vi "CSM - All Relationships of Broadcast Registry.vi"() -> ()   [LabVIEW 2017, in "Communicable State Machine.lvlib"]
uses:
  Communicable State Machine.lvlib
  CSM - Broadcast Message Type.ctl
  _Support/FGV-BroadcastRegistry/global-CSMQ FGV Change Flag.vi
  _Support/CSMQ/_CSMOFGV.vi
panel:
  out "error out":errorcluster
  in  "error in (no error)":errorcluster
  out "Array":T2(array[cluster])
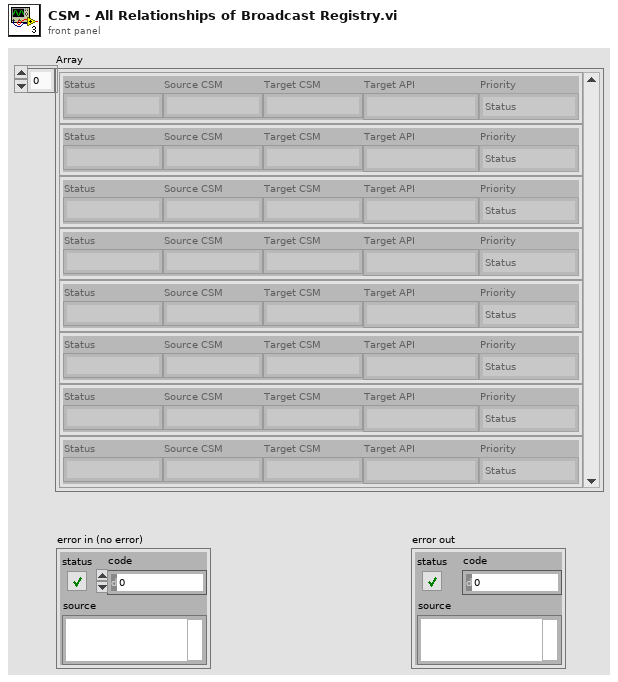
[diagram p1: front panel]
types:
  T1 = typedef "Communicable State Machine.lvlib/CSM - Broadcast Message Type.ctl" = enum16{"Status", "Interrupt(High)"}
  T2 = cluster{"Status":string, "Source CSM":string, "Target CSM":string, "Target API":string, "Priority":T1}[]
  T3 = cluster{"Target CSM":string, "Target State":string, "Priority":T1}[]
  T4 = cluster{"Status":string, "Source CSM":string, "Target CSM":string, "Target API":string, "Priority":T1}
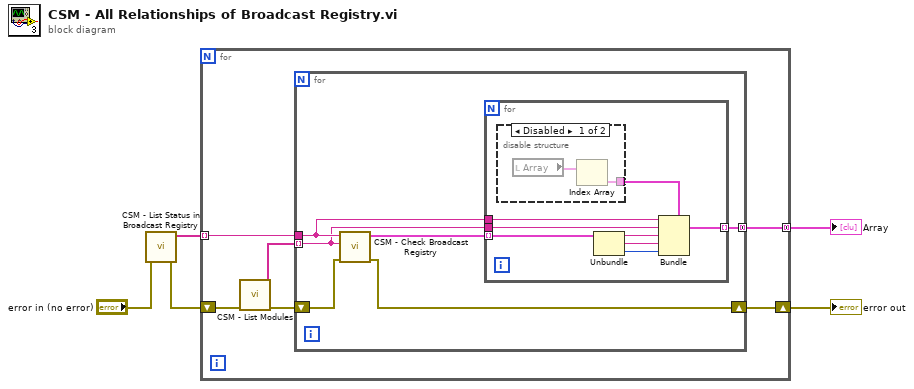
[diagram p0: block diagram]
diagram:
  n1 = call "CSM - List Status in Broadcast Registry.vi"("error in (no error)"="error in (no error)") -> ("error out"=w2:errorcluster, "Status in Registry"=w5:string[])  [unwired: 9 in]
  n2 = for {
    tunnel: w5 -> [w11] mode=indexing
    tunnel: [w9] -> w4 mode=concatenating
    shift-right: [w6] -> w1
    shift-left: w2 -> [w8]
    n3 = call "CSM - List Modules.vi"("Error in"=w8) -> ("Error out"=w7:errorcluster, "Module Names"=w10:string[])  [unwired: 9 in]
    n4 = for {
      tunnel: w11 -> [w17]
      tunnel: w10 -> [w15] mode=indexing
      tunnel: [w14] -> w9 mode=concatenating
      shift-right: [w12] -> w6
      shift-left: w7 -> [w13]
      n5 = call "CSM - Check Broadcast Registry.vi"("error in (no error)"=w13, "CSM Name"=w15, "Broadcast state"=w17) -> ("error out"=w12:errorcluster, "Array"=w16:T3)  [unwired: 7 in]
      n6 = for {
        tunnel: w17 -> [w25]
        tunnel: w16 -> [w22] mode=indexing
        tunnel: w15 -> [w24]
        tunnel: [w23] -> w14 mode=indexing
        n7 = disable-structure shown="Disabled" {
          disable-tunnel: [w26 _] -> w18
          frame Disabled {
            n8 = local read "Array"() -> (w27:T2)
            n9 = Index Array(array=w27) -> (element=w26:T4)  [unwired: 1 in]
          }
          frame Enabled {
          }
        }
        n10 = Unbundle(w22) -> ("Target CSM"=w21:string, "Target State"=w20:string, "Priority"=w19:T1)
        n11 = Bundle(cluster=w18, "Status"=w25, "Source CSM"=w24, "Target CSM"=w21, "Target API"=w20, "Priority"=w19) -> (w23:T4)
      }
    }
  }
  "Array" <- w4
  "error out" <- w1
